vi "_Open.vi"(8 "error in":errorcluster, 10 "Serial Number":i32, 11 "Device In":i32) -> (0 "error out":errorcluster, 3 "Device Out":i32)   [LabVIEW 2014]
uses:
  phidget21.dll
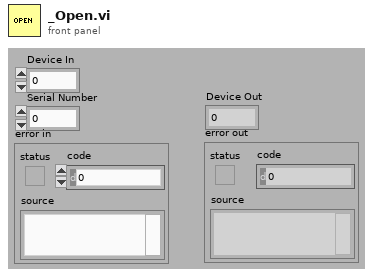
[diagram p1: front panel]
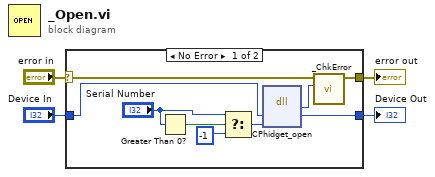
[diagram p0: block diagram]
diagram:
  n1 = case shown="No Error" "error in" {
    selector: "error in" -> [w7 w15]
    tunnel: [w5 w15] -> w3
    tunnel: [w9 w14] -> w2
    tunnel: "Device In" -> [w8 w14]
    frame No Error {
      n2 = Greater Than 0?(x="Serial Number") -> (x > 0?=w13:bool)
      n3 = Select(t="Serial Number", s=w13, f=-1 ("t")) -> (s? t:f=w12:i32)
      n4 = dll-call lib="phidget21.*" fn="CPhidget_open"("phid"=w8, "serialNumber"=w12) -> (w6:i32, "phid"=w9:i32)  [unwired: 4 in, 2 out]
      n5 = call "_ChkError.vi"("Return Code"=w6, "error in (no error)"=w7) -> ("error out"=w5:errorcluster)  [unwired: 9 in]
    }
    frame Error {
    }
  }
  "error out" <- w3
  "Device Out" <- w2
